vi "Statement - fields.vi"(8 "error in (no error)":errorcluster) -> (0 "error out":errorcluster)   [LabVIEW 2026, in "Tests.lvlib"]
doc: "Integration test (Caraya). Verifies a statement logged through the Logger reaches a single registered appender. Launches a manager with the default file disabled and a queue-mode relay capture probe (Open Test Mgr), logs one INFO statement, dequeues from the capture queue with a timeout, and asserts it was delivered and its message matches. Tears down with Close Test Mgr regardless of assertion outcome (SRS-LMBR-019). Uses the manager fixture; no temp root needed.\n\nImplements LMBR-T-029 -> SRS-019. Assert-level IDs: Test-ID-Assert-Checklist.md."
uses:
  Tests.lvlib
  src/TypeDefs/Severity.ctl
  <vilib>/addons/_JKI Toolkits/Caraya/classes/Assert/Assert Equal Value_Variant.vi
  <vilib>/addons/_JKI Toolkits/Caraya/classes/Assert/Assert True.vi
  <vilib>/addons/_JKI Toolkits/Caraya/classes/Test/Test.lvclass
  src/Lumberjack.lvlib
  src/Public/Logger.lvclass/Logger.lvclass
  <vilib>/addons/_JKI Toolkits/Caraya/classes/Assert/Assert.lvclass
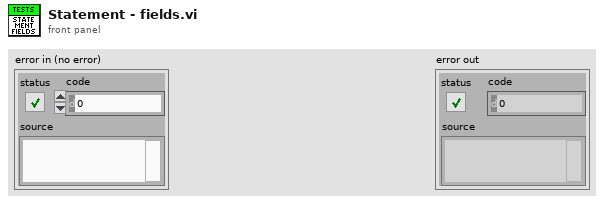
[diagram p1: front panel]
types:
  T1 = typedef "Lumberjack.lvlib/Severity.ctl" = enum16{"OFF", "FATAL", "ERROR", "WARN", "INFO", "DEBUG", "TRACE", "ALL"}
  T2 = typedef "Lumberjack.lvlib/Statement.ctl" = cluster{"timestamp":timestamp, "level":T1, "sourceTag":string, "originVI":string, "message":string}
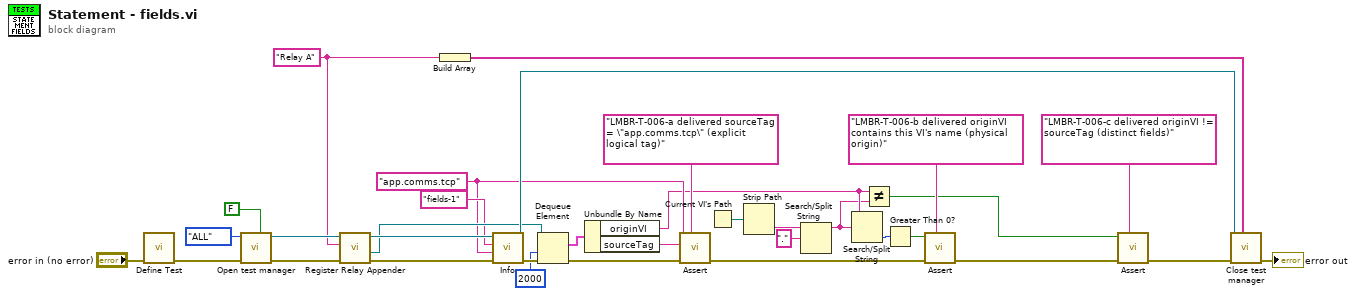
[diagram p0: block diagram]
diagram:
  w15 = "app.comms.tcp" ("sourceTag")
  w22 = "Relay A" ("id in")
  n1 = call <vilib>:"Define Test.vi"("error in (no error)"="error in (no error)") -> ("error out"=w33:errorcluster)  [unwired: 9 in, 1 out]
  n2 = call "Open test manager.vi"("enableDefaultFile"=FALSE, "error in (no error)"=w33, "globalThreshold"=Severity."ALL") -> ("error out"=w26:errorcluster, "Logger out"=w27:refnum<class "Logger.lvclass">)  [unwired: 7 in]
  n3 = call "Register Relay Appender.vi"("error in (no error)"=w26, "id in"=w22, "Logger in"=w27) -> ("error out"=w24:errorcluster, "relayQueue"=w23:refnum<queue>, "Logger out"=w25:refnum<class "Logger.lvclass">)  [unwired: 5 in, 1 out]
  n4 = Build Array(w22) -> (w20:string[])
  n5 = call "Info.vi"("error in (no error)"=w24, "sourceTag"=w15, "message"="fields-1", "Logger in"=w25) -> ("error out"=w31:errorcluster, "Logger out"=w28:refnum<class "Logger.lvclass">)  [unwired: 6 in]
  n6 = Dequeue Element(queue=w23, timeout in ms (-1)=2000, error in (no error)=w31) -> (element=w29:T2, error out=w19:errorcluster)  [unwired: 2 out]
  n7 = Unbundle By Name(w29) -> ("originVI"=w6:string, "sourceTag"=w17:string)
  n8 = call-poly <vilib>:"Assert.vi"("Label"="LMBR-T-006-a delivered sourceTag = \"app.comms.tcp\" (explicit logical tag)", "error in (no error)"=w19, "Actual"=w17, "Expected"=w15) -> ("error out"=w9:errorcluster)  [unwired: 6 in, 1 out]
  n9 = Current VI's Path() -> (path=w13:path)
  n10 = Strip Path(path=w13) -> (name=w12:string)  [unwired: 1 out]
  n11 = Search/Split String(string=w12, search string/char (-)=".") -> (substring before match=w5:string)  [unwired: 1 in, 2 out]
  n12 = Search/Split String(string=w6, search string/char (-)=w5) -> (offset of match=w8:i32)  [unwired: 1 in, 2 out]
  n13 = Not Equal?(x=w6, y=w5) -> (x != y?=w1:bool)
  n14 = Greater Than 0?(x=w8) -> (x > 0?=w7:bool)
  n15 = call-poly <vilib>:"Assert.vi"("Label"="LMBR-T-006-b delivered originVI contains this VI's name (physical origin)", "error in (no error)"=w9, "True?"=w7) -> ("error out"=w3:errorcluster)  [unwired: 7 in, 1 out]
  n16 = call-poly <vilib>:"Assert.vi"("Label"="LMBR-T-006-c delivered originVI != sourceTag (distinct fields)", "error in (no error)"=w3, "True?"=w1) -> ("error out"=w2:errorcluster)  [unwired: 7 in, 1 out]
  n17 = call "Close test manager.vi"("queueIDList"=w20, "error in (no error)"=w2, "Logger in"=w28) -> ("error out"=→"error out":errorcluster)  [unwired: 6 in]
